vi "add_PoseWithCovariance_roslv.vi"(4 "PoseCovariance":T1={"Pose"={"Point"={"x"=0.0, "y"=0.0, "z"=0.0}, "Quaternion"={"x"=0.0, "y"=0.0, "z"=0.0, "w"=0.0}}, "Covariance"=[0.0, 0.0, 0.0, 0.0, 0.0]}, 5 "msg in":string) -> (2 "msg out":string)   [LabVIEW 2014]
doc: "Flattens a pose with covariance into a message"
uses:
  std_msgs/subs/float64Array_roslv.vi
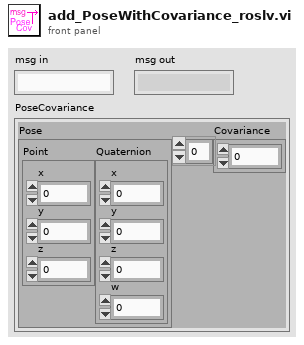
[diagram p1: front panel]
types:
  T1 = cluster{"Pose":cluster{"Point":cluster{"x":dbl, "y":dbl, "z":dbl}, "Quaternion":cluster{"x":dbl, "y":dbl, "z":dbl, "w":dbl}}, "Covariance":dbl[]}
  T2 = cluster{"Point":cluster{"x":dbl, "y":dbl, "z":dbl}, "Quaternion":cluster{"x":dbl, "y":dbl, "z":dbl, "w":dbl}}
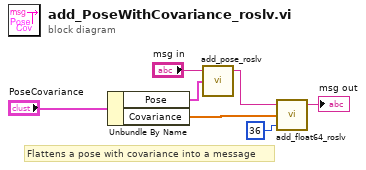
[diagram p0: block diagram]
diagram:
  # "Flattens a pose with covariance into a message"
  n1 = Unbundle By Name("PoseCovariance") -> ("Pose"=w2:T2, "Covariance"=w1:dbl[])
  n2 = call "add_pose_roslv.vi"("Pose"=w2, "msg in"="msg in") -> ("msg out"=w4:string)  [unwired: 3 in]
  n3 = call-poly "add_float64_roslv.vi"("Array Length"=36, "Array"=w1, "msg in"=w4) -> ("msg out"=→"msg out":string)  [unwired: 2 in]
